vi "Inverse Kinematics with DH.vi"(4 "Initial guess":dbl[](array[numeric])=[-1.0, -1.0, -1.0, -1.0], 6 "Joint Limits":dbl[][](array[numeric])=[[-68.0, -4.0], [-26.0, 52.0], [-40.0, 23.0], [-180.0, 180.0]] format="%#.3g", 7 "armID":i32=1, 8 "z":dbl, 9 "y":dbl, 10 "x":dbl, 11 "toolInsertionOffset":dbl=-54.76) -> (0 "j4":dbl, 1 "j3":dbl, 2 "j2":dbl, 3 "j1":dbl)   [LabVIEW 2016]
uses:
  RobotKinematicsDLL.dll
panel:
  out "return type":i32
  out "appended array":dbl[](array[numeric])
  out "error IO":errorcluster
  out "KINEMATICS_RET_SOLUTION_BEYOND_LIMIT":bool
  out "KINEMATICS_RET_NO_SOLUTION":bool
  out "KINEMATICS_RET_WRONG_ARM_ID":bool
  # ">>"
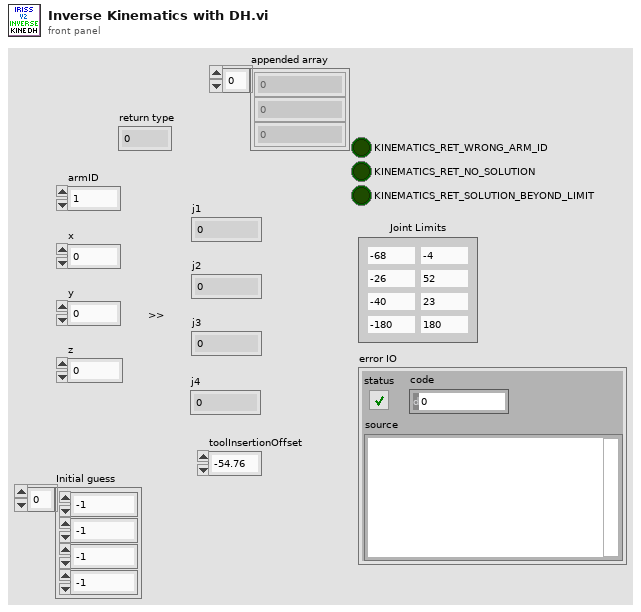
[diagram p1: front panel]
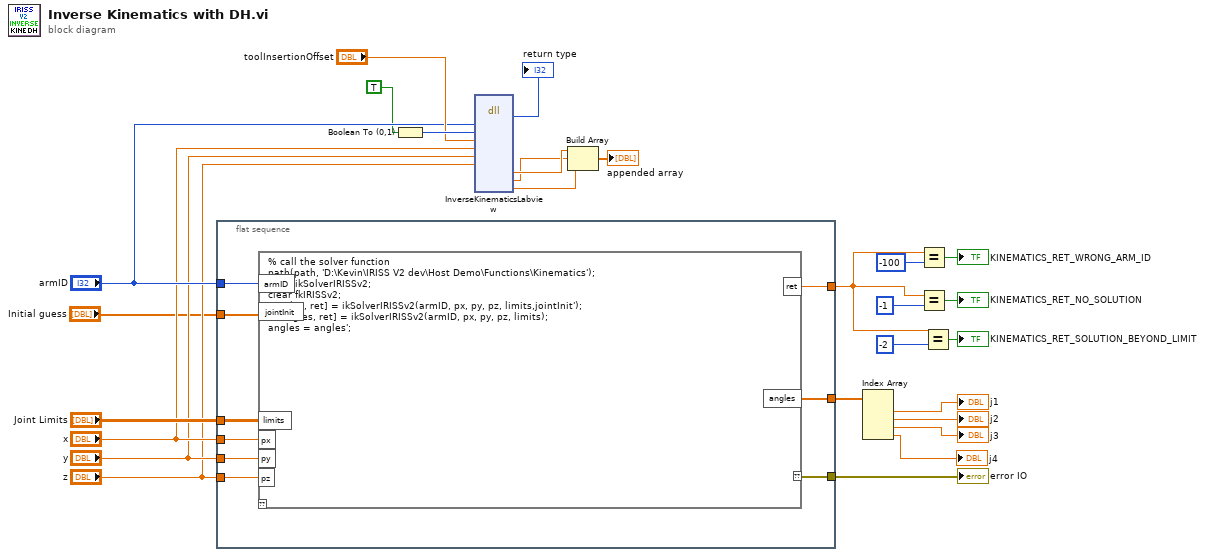
[diagram p0: block diagram]
diagram:
  n1 = flat-sequence {
    tunnel: [w33] -> w27
    tunnel: "y" -> [w36]
    tunnel: "x" -> [w35]
    tunnel: "z" -> [w34]
    tunnel: "armID" -> [w30]
    tunnel: [w32] -> w23
    tunnel: [w31] -> w15
    tunnel: "Joint Limits" -> [w29]
    tunnel: "Initial guess" -> [w28]
    frame #0 {
      n2 = script code="% call the solver function\npath(path, 'D:\\Kevin\\IRISS V2 dev\\Host Demo\\Functions\\Kinematics');\nclear ikSolverIRISSv2;\nclear fkIRISSv2;\n[angles, ret] = ikSolverIRISSv2(armID, px, py, pz, limits,jointInit');\n%[angles, ret] = ikSolverIRISSv2(armID, px, py, pz, limits);\nangles = angles';"("px"=w35, "py"=w36, "pz"=w34, "armID"=w30, "limits"=w29, "jointInit"=w28) -> ("??"=w32:errorcluster, "angles"=w33:dbl[], "ret"=w31:dbl)  [unwired: 1 in]
    }
  }
  n3 = Boolean To (0,1)(Boolean=TRUE) -> (0, 1=w14:i16)
  n4 = dll-call lib="D:/Kevin/IRISS V2 dev/Host Demo/Functions/RobotKinematicsDLL.dll" fn="InverseKinematicsLabview"("id"="armID", "isToolInsideEye"=w14, "toolInsertionOffset"="toolInsertionOffset", "x"="x", "y"="y", "z"="z") -> ("return type"=→"return type":i32, "j1"=w6:dbl, "j2"=w5:dbl, "j3"=w4:dbl)  [unwired: 12 in, 2 out]
  n5 = Build Array(w6, w5, w4) -> (→"appended array":dbl[])
  n6 = Index Array(array=w27) -> (element #1=→"j1":dbl, element #2=→"j2":dbl, element #3=→"j3":dbl, element #4=→"j4":dbl)  [unwired: 4 in]
  n7 = Equal?(x=w15, y=-100) -> (x = y?=→"KINEMATICS_RET_WRONG_ARM_ID":bool)
  n8 = Equal?(x=w15, y=-1) -> (x = y?=→"KINEMATICS_RET_NO_SOLUTION":bool)
  n9 = Equal?(x=w15, y=-2) -> (x = y?=→"KINEMATICS_RET_SOLUTION_BEYOND_LIMIT":bool)
  "error IO" <- w23
